vi "manual-induction-furnace-control.vi"() -> ()   [LabVIEW 2019]
uses:
  <vilib>/DAQmx/read.llb/DAQmx Read (Analog 2D DBL NChan NSamp).vi
  <vilib>/Analysis/baseanly.llb/Mean (DBL).vi
  <vilib>/DAQmx/read.llb/DAQmx Read (Analog 1D DBL 1Chan NSamp).vi
  <vilib>/DAQmx/write.llb/DAQmx Write (Analog DBL 1Chan 1Samp).vi
  <vilib>/DAQmx/create/channels.llb/DAQmx Create Channel (AO-Current-Basic).vi
  <vilib>/DAQmx/create/channels.llb/DAQmx Create Channel (AI-Current-Basic).vi
  <vilib>/DAQmx/create/channels.llb/DAQmx Create Channel (AI-Voltage-Basic).vi
  <vilib>/DAQmx/miscellaneous.llb/DAQmx Fill In Error Info.vi
  <vilib>/Analysis/NI_AALBase.lvlib
panel:
  in  "Furnace Enable":bool
  in  "Furnace Stop":bool
  out "Valve Output":dbl format="%#_3g"
  in  "Main State":enum16{"IDLE", "TIMER"}(ring)
  in  "DONE":bool
  in  "ESTOP":bool
  in  "Valve Open":bool
  in  "Purge Flow On":bool
  out "Pressure":dbl format="%#_3g"
  in  "Tab Control":T1(tab)
  in  "Start Test":bool
  in  "Test Settings":bool
  in  "Error Email":string
  in  "Power Input":dbl
  in  "Start Hold":bool
  in  "Argon Out":dbl format="%#_4g"
  out "Test Time Remaining":string
  out "End Result":string
  in  "Temperature Drop Limit":dbl=60.0
  in  "Pressure Limit":dbl=0.002
  in  "Time to Hold":dbl=480.0
  in  "Finish Editting":bool
  out "Temperature":dbl format="%#_5g"
  out "Power Out":dbl
  # "%"
  # "°C"
  # "Torr"
  # "To start this test make sure your test settings are confirmed by looking at the test settings before pressing the start test below. If an error occurs during the test, the code will stop the furnace then display a window explaining why the test was stopped."
  # "This is a manual control window. Slowly increment the power percentage below from 10% to your desired power while monitoring the temperature. Between each time you increment the power allow enough time for the item in the furnace to come to equilibrium before increasing the power more. Press the Start Hold button once you reach your desired power."
  # "%"
  # "%"
  # "This is the amount of time that is left for your test on the furnace"
  # "Your test has been stopped. Below you can see if the test finished successfully or if an error occurred."
  # "min"
  # "Torr"
  # "°C"
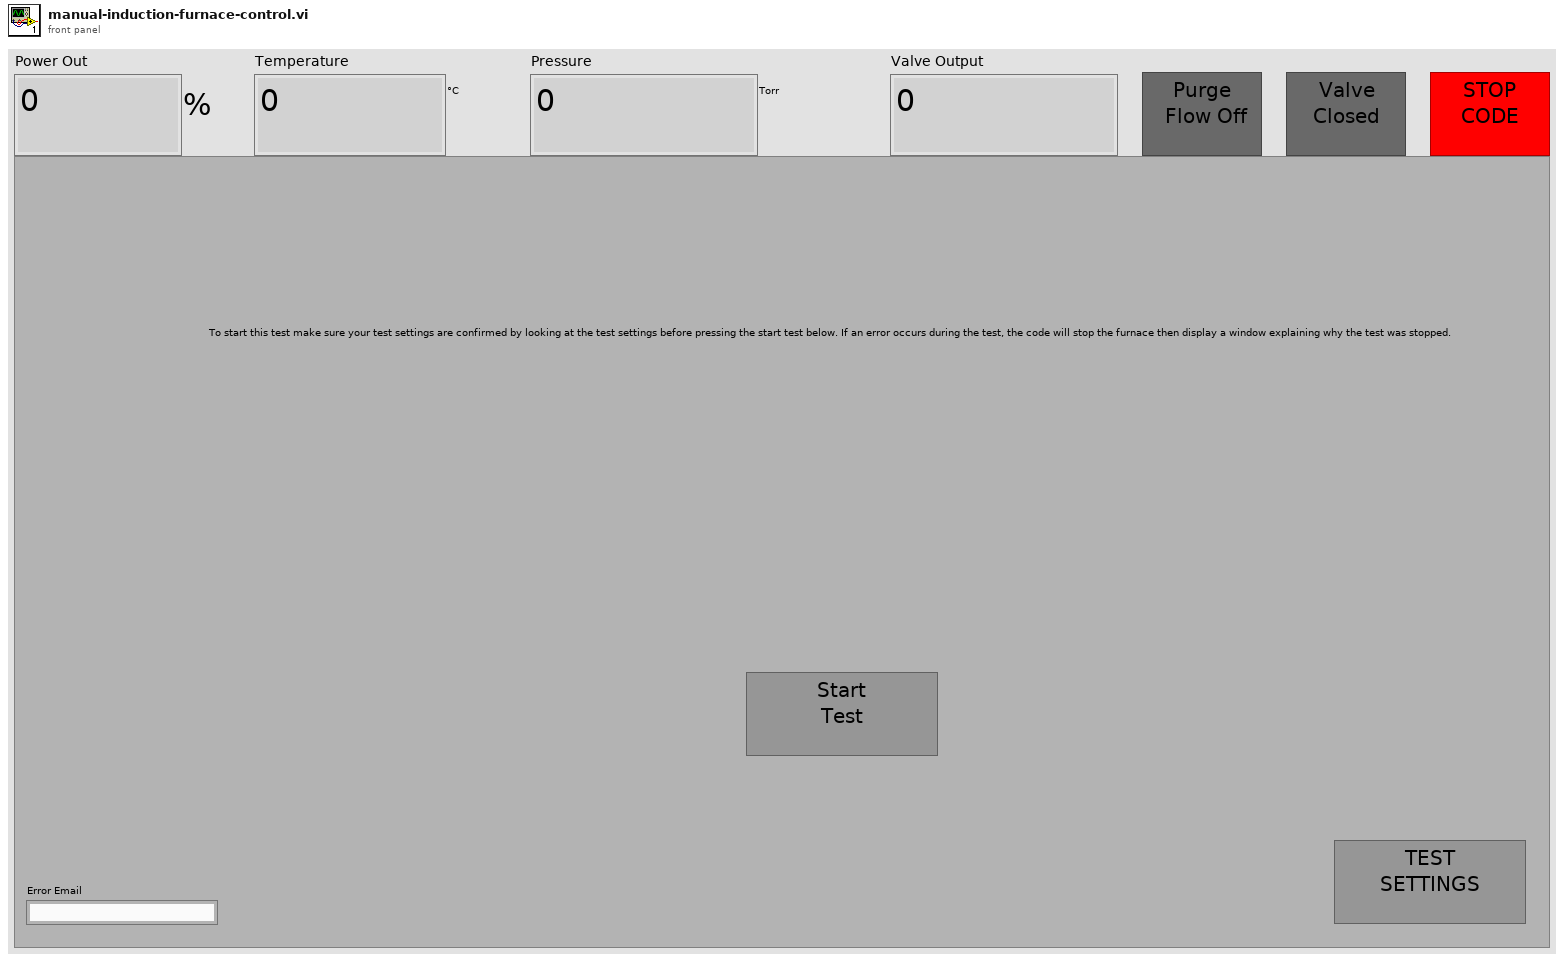
[diagram p1: front panel]
types:
  T1 = enum32{"Start", "Manual Control", "Timer", "End", "Settings"}
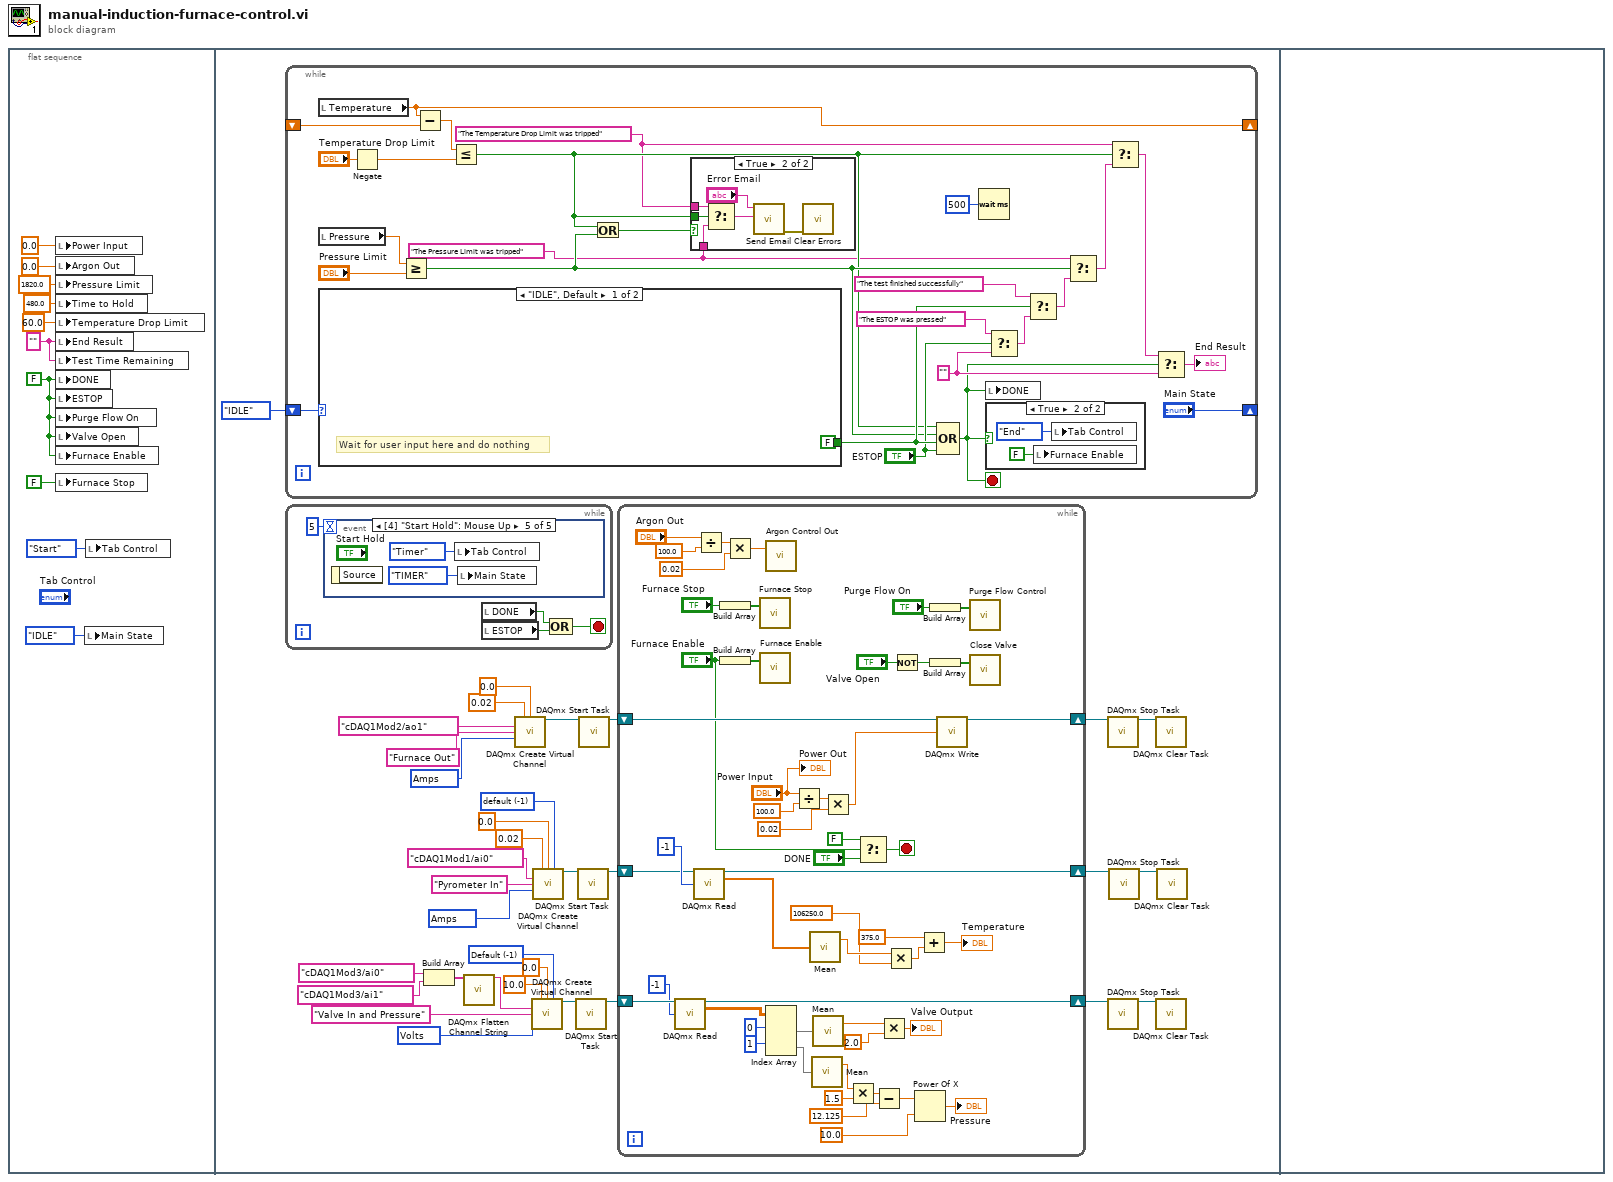
[diagram p0: block diagram]
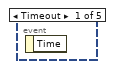
[diagram p2: hidden frame]
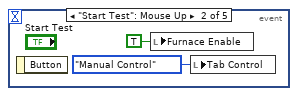
[diagram p3: hidden frame]
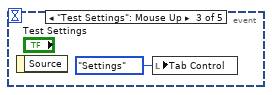
[diagram p4: hidden frame]
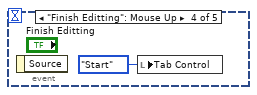
[diagram p5: hidden frame]
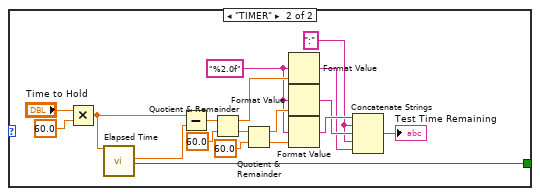
[diagram p8: hidden frame]
diagram:
  n1 = flat-sequence {
    frame #0 {
      w9 = "" ("End Result")
      w6 = FALSE
      n2 = local write "Power Input"(0.0 ("Power Input")) -> ()
      n3 = local write "Argon Out"(0.0 ("Pressure Limit")) -> ()
      n4 = local write "Pressure Limit"(1820.0 ("Pressure Limit")) -> ()
      n5 = local write "Time to Hold"(480.0 ("Time to Hold")) -> ()
      n6 = local write "Temperature Drop Limit"(60.0 ("Time to Hold")) -> ()
      n7 = local write "End Result"(w9) -> ()
      n8 = local write "Test Time Remaining"(w9) -> ()
      n9 = local write "DONE"(w6) -> ()
      n10 = local write "ESTOP"(w6) -> ()
      n11 = local write "Purge Flow On"(w6) -> ()
      n12 = local write "Valve Open"(w6) -> ()
      n13 = local write "Furnace Enable"(w6) -> ()
      n14 = local write "Furnace Stop"(FALSE) -> ()
      n15 = local write "Main State"(enum16{"IDLE", "TIMER", "END"}."IDLE" ("Main State")) -> ()
      n16 = local write "Tab Control"(T1."Start" ("Tab Control")) -> ()
    }
    frame #1 {
      w19 = 10348 items=["Volts"=10348, "From Custom Scale"=10065] ("units")
      w21 = -1 items=["Default"=-1, "RSE"=10083, "NRSE"=10078, "Differential"=10106, "Pseudodifferential"=12529] ("input terminal configuration")
      w32 = -1 items=["default"=-1, "RSE"=10083, "NRSE"=10078, "Differential"=10106, "Pseudodifferential"=12529] ("input terminal configuration")
      w18 = 10342 items=["Amps"=10342, "From Custom Scale"=10065] ("units")
      w37 = 10342 items=["Amps"=10342, "From Custom Scale"=10065] ("units")
      n17 = while {
        shift-right: ["Main State"] -> _
        shift-left: enum16{"IDLE", "TIMER"}."IDLE" -> [w130]
        shift-right: [w126] -> _
        shift-left: _ -> [w125]
        stop <- w111 stop-if-true
        w115 = "" ("End Result")
        w105 = "The Pressure Limit was tripped" ("End Result")
        w106 = "The Temperature Drop Limit was tripped" ("End Result")
        n18 = local read "Temperature"() -> (w126:dbl)
        n19 = local read "Pressure"() -> (w128:dbl)
        n20 = case shown="\"IDLE\", Default" w130 {
          tunnel: [FALSE w155] -> w121
          frame "IDLE", Default {
            # "Wait for user input here and do nothing"
          }
          frame "TIMER" {
            w142 = ":" ("string")
            w145 = "%2.0f" ("format string")
            n21 = Multiply(x="Time to Hold", y=60.0) -> (x*y=w153:dbl)
            n22 = call "Elapsed Time"("Time Target (s)"=w153) -> ("Elapsed Time (s)"=w154:dbl, "Time has Elapsed"=w155:bool)  [unwired: 11 in, 6 out]
            n23 = Subtract(x=w153, y=w154) -> (x-y=w152:dbl)
            n24 = Quotient & Remainder(x=w152, y=60.0) -> (x-y*floor(x/y)=w148:dbl, floor(x/y)=w150:dbl)
            n25 = Quotient & Remainder(x=w150, y=60.0) -> (x-y*floor(x/y)=w146:dbl, floor(x/y)=w147:dbl)
            n26 = Format Value(format string=w145, value (0)=w148) -> (output string=w141:string)  [unwired: 1 in]
            n27 = Format Value(format string=w145, value (0)=w146) -> (output string=w143:string)  [unwired: 1 in]
            n28 = Format Value(format string=w145, value (0)=w147) -> (output string=w144:string)  [unwired: 1 in]
            n29 = Concatenate Strings(w144, w142, w143, w142, w141) -> (→"Test Time Remaining":string)
          }
        }
        n30 = Negate(x="Temperature Drop Limit") -> (-x=w123:dbl)
        n31 = Greater Or Equal?(x=w128, y="Pressure Limit") -> (x >= y?=w109:bool)
        n32 = Subtract(x=w126, y=w125) -> (x-y=w122:dbl)
        n33 = Less Or Equal?(x=w122, y=w123) -> (x <= y?=w107:bool)
        n34 = Or(x=w107, y=w109) -> (x .or. y?=w108:bool)
        n35 = case shown="True" w108 {
          tunnel: w107 -> [_ w136]
          tunnel: w106 -> [_ w135]
          tunnel: w105 -> [_ w134]
          frame False {
          }
          frame True {
            n36 = Select(t=w135, s=w136, f=w134) -> (s? t:f=w133:string)
            n37 = call "Send Email.vi"("Message"=w133, "Recipient Email"="Error Email") -> ("error out"=w131:errorcluster)  [unwired: 9 in]
            n38 = call <vilib>:"Clear Errors.vi"("error in (no error)"=w131) -> ()  [unwired: 5 in, 2 out]
          }
        }
        n39 = Compound Arithmetic op=OR(w107, w109, w121, "ESTOP") -> (w111:bool)
        n40 = Wait (ms)(milliseconds to wait=u32 500) -> ()  [unwired: 1 out]
        n41 = local write "DONE"(w111) -> ()
        n42 = case shown="True" w111 {
          frame False {
          }
          frame True {
            n43 = local write "Furnace Enable"(FALSE ("Furnace Enable")) -> ()
            n44 = local write "Tab Control"(T1."End" ("Tab Control")) -> ()
          }
        }
        n45 = Select(t="The ESTOP was pressed" ("End Result"), s="ESTOP", f=w115) -> (s? t:f=w118:string)
        n46 = Select(t="The test finished successfully" ("End Result"), s=w121, f=w118) -> (s? t:f=w119:string)
        n47 = Select(t=w105, s=w109, f=w119) -> (s? t:f=w114:string)
        n48 = Select(t=w106, s=w107, f=w114) -> (s? t:f=w113:string)
        n49 = Select(t=w113, s=w111, f=w115) -> (s? t:f=→"End Result":string)
      }
      n50 = while {
        stop <- w46 stop-if-true
        n51 = event shown="[4] \"Start Hold\": Mouse Up" {
          selector: _ -> [_ _ _ _ _]
          dyn-events: _ -> [_ _ _ _ _]
          timeout: 5 -> [_ _ _ _ _]
          event Timeout {
            n52 = event-data() -> ()  [unwired: 1 in, 1 out]
          }
          event "Start Test": Mouse Up {
            n53 = event-data() -> ()  [unwired: 1 in, 1 out]
            n54 = local write "Furnace Enable"(TRUE ("Furnace Enable")) -> ()
            n55 = local write "Tab Control"(T1."Manual Control" ("Tab Control")) -> ()
          }
          event "Test Settings": Mouse Up {
            n56 = event-data() -> ()  [unwired: 1 in, 1 out]
            n57 = local write "Tab Control"(T1."Settings" ("Tab Control")) -> ()
          }
          event "Finish Editting": Mouse Up {
            n58 = event-data() -> ()  [unwired: 1 in, 1 out]
            n59 = local write "Tab Control"(T1."Start" ("Tab Control")) -> ()
          }
          event "Start Hold": Mouse Up {
            n60 = event-data() -> ()  [unwired: 1 in, 1 out]
            n61 = local write "Tab Control"(T1."Timer" ("Tab Control")) -> ()
            n62 = local write "Main State"(enum16{"IDLE", "TIMER"}."TIMER" ("Main State")) -> ()
          }
        }
        n63 = local read "DONE"() -> (w45:bool)
        n64 = local read "ESTOP"() -> (w47:bool)
        n65 = Compound Arithmetic op=OR(w45, w47) -> (w46:bool)
      }
      n66 = Build Array(tag "cDAQ1Mod3/ai0" ("physical channels"), tag "cDAQ1Mod3/ai1" ("physical channels")) -> (w12:tag[])
      n67 = call <vilib>:"DAQmx Flatten Channel String.vi"("names in"=w12) -> ("names out"=w11:string)  [unwired: 13 in, 1 out]
      n68 = call-poly <vilib>:"DAQmx Create Virtual Channel.vi"("maximum value"=0.02, "minimum value"=0.0, "physical channels"=tag "cDAQ1Mod2/ao1", "name to assign"="Furnace Out", "units"=w37) -> ("task out"=w38:refnum<k21>)  [unwired: 9 in, 1 out]
      n69 = call-poly <vilib>:"DAQmx Create Virtual Channel.vi"("maximum value"=10.0, "minimum value"=0.0, "input terminal configuration"=w21, "physical channels"=w11, "name to assign"="Valve In and Pressure", "units"=w19) -> ("task out"=w24:refnum<k21>)  [unwired: 8 in, 1 out]
      n70 = call-poly <vilib>:"DAQmx Create Virtual Channel.vi"("maximum value"=0.02, "minimum value"=0.0, "input terminal configuration"=w32, "physical channels"=tag "cDAQ1Mod1/ai0", "name to assign"="Pyrometer In", "units"=w18) -> ("task out"=w31:refnum<k21>)  [unwired: 8 in, 1 out]
      n71 = call <vilib>:"DAQmx Start Task.vi"("task/channels in"=w24) -> ("task out"=w17:refnum<k21>)  [unwired: 13 in, 1 out]
      n72 = call <vilib>:"DAQmx Start Task.vi"("task/channels in"=w31) -> ("task out"=w30:refnum<k21>)  [unwired: 13 in, 1 out]
      n73 = call <vilib>:"DAQmx Start Task.vi"("task/channels in"=w38) -> ("task out"=w29:refnum<k21>)  [unwired: 13 in, 1 out]
      n74 = while {
        shift-right: [w81] -> w25
        shift-left: w29 -> [w83]
        shift-right: [w84] -> w27
        shift-left: w30 -> [w86]
        shift-right: [w74] -> w15
        shift-left: w17 -> [w76]
        stop <- w77 stop-if-true
        n75 = call-poly <vilib>:"DAQmx Read.vi"("task/channels in"=w76, "number of samples per channel"=-1) -> ("task out"=w74:refnum<k21>, "data"=w65:dbl[][])  [unwired: 11 in, 1 out]
        n76 = call-poly <vilib>:"DAQmx Read.vi"("task/channels in"=w86, "number of samples per channel"=-1) -> ("task out"=w84:refnum<k21>, "data"=w87:dbl[])  [unwired: 11 in, 1 out]
        n77 = Divide(x="Argon Out", y=100.0) -> (x/y=w58:dbl)
        n78 = Build Array("Furnace Stop") -> (w100:bool[])
        n79 = Build Array("Furnace Enable") -> (w101:bool[])
        n80 = Multiply(x=w58, y=0.02) -> (x*y=w54:dbl)
        n81 = call "Furnace Stop"("data"=w100) -> ()  [unwired: 17 in, 2 out]
        n82 = call "Furnace Enable"("data"=w101) -> ()  [unwired: 17 in, 2 out]
        n83 = call "Argon Control Out"("data"=w54) -> ()  [unwired: 17 in, 2 out]
        n84 = Index Array(array=w65, index (row) #1=0 ("index (row)"), index (row) #2=1 ("index (row)")) -> (element #1=w62:dbl[], element #2=w61:dbl[])  [unwired: 2 in]
        n85 = Divide(x="Power Input", y=100.0) -> (x/y=w94:dbl)
        n86 = call-poly <vilib>:"Mean.vi"("X"=w87) -> ("mean"=w91:dbl)  [unwired: 1 out]
        n87 = call-poly <vilib>:"Mean.vi"("X"=w61) -> ("mean"=w73:dbl)  [unwired: 1 out]
        n88 = call-poly <vilib>:"Mean.vi"("X"=w62) -> ("mean"=w66:dbl)  [unwired: 1 out]
        n89 = Multiply(x=w94, y=0.02) -> (x*y=w82:dbl)
        n90 = Multiply(x=w73, y=1.5) -> (x*y=w71:dbl)
        n91 = Select(t=FALSE, s="Furnace Enable", f="DONE") -> (s? t:f=w77:bool)
        n92 = Subtract(x=w71, y=12.125) -> (x-y=w69:dbl)
        n93 = Multiply(x=w66, y=2.0) -> (x*y=→"Valve Output":dbl)
        n94 = Multiply(x=w91, y=106250.0) -> (x*y=w90:dbl)
        n95 = Not(x="Valve Open") -> (.not. x?=w59:bool)
        n96 = Power Of X(1:10.0 ("x"), 2:w69) -> (0:→"Pressure":dbl)
        n97 = Add(x=375.0, y=w90) -> (x+y=→"Temperature":dbl)
        n98 = Build Array("Purge Flow On") -> (w98:bool[])
        n99 = Build Array(w59) -> (w97:bool[])
        n100 = call-poly <vilib>:"DAQmx Write.vi"("task/channels in"=w83, "data"=w82) -> ("task out"=w81:refnum<k21>)  [unwired: 11 in, 2 out]
        n101 = call "Purge Flow Control"("data"=w98) -> ()  [unwired: 17 in, 2 out]
        n102 = call "Close Valve"("data"=w97) -> ()  [unwired: 17 in, 2 out]
        "Power Out" <- "Power Input"
      }
      n103 = call <vilib>:"DAQmx Stop Task.vi"("task/channels in"=w25) -> ("task out"=w26:refnum<k21>)  [unwired: 13 in, 1 out]
      n104 = call <vilib>:"DAQmx Stop Task.vi"("task/channels in"=w15) -> ("task out"=w16:refnum<k21>)  [unwired: 13 in, 1 out]
      n105 = call <vilib>:"DAQmx Stop Task.vi"("task/channels in"=w27) -> ("task out"=w28:refnum<k21>)  [unwired: 13 in, 1 out]
      n106 = call <vilib>:"DAQmx Clear Task.vi"("task in"=w26) -> ()  [unwired: 14 in, 1 out]
      n107 = call <vilib>:"DAQmx Clear Task.vi"("task in"=w16) -> ()  [unwired: 14 in, 1 out]
      n108 = call <vilib>:"DAQmx Clear Task.vi"("task in"=w28) -> ()  [unwired: 14 in, 1 out]
    }
    frame #2 {
    }
  }
